vi "NoItemsFound.vi"(8 "error in (no error)":errorcluster, 11 "ExecuteMultipleBuildSpecs in":refnum<class "ExecuteMultipleBuildSpecs.lvclass">) -> (2 "CLI Process Return Code":i32, 3 "ExecuteMultipleBuildSpecs out":refnum<class "ExecuteMultipleBuildSpecs.lvclass">)   [LabVIEW 2020, in "ExecuteMultipleBuildSpecs.lvclass"]
doc: "Sets the LabVIEWCLI exit code if no build specs matching the criteria are found in the project."
uses:
  ExecuteMultipleBuildSpecs.lvclass
  Program Files (x86)/National Instruments/Shared/LabVIEW CLI/Operations/CoreOperation/CoreOperation.lvclass
  Program Files (x86)/National Instruments/Shared/LabVIEW CLI/Operations/Utilities/Logger/Logger.lvclass
  C:/Program Files (x86)/National Instruments/Shared/LabVIEW CLI/Operations/CoreOperation/CoreOperation.lvclass
  C:/Work/1_New Activities/JenkinsTest/BuildSystem/lv/operations/ExecuteMultipleBuildSpecs/ExecuteMultipleBuildSpecs.lvclass
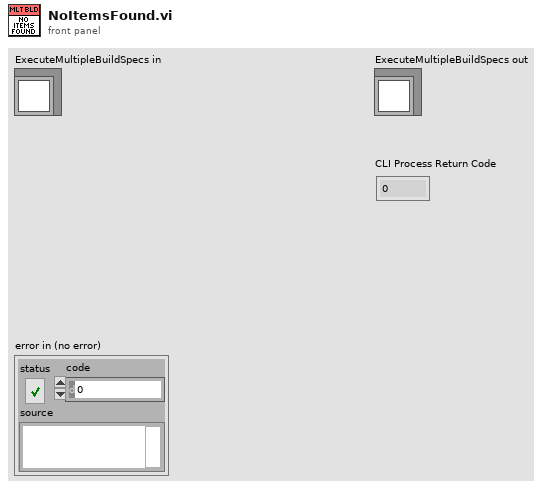
[diagram p1: front panel]
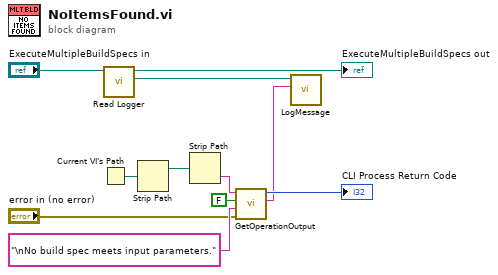
[diagram p0: block diagram]
diagram:
  n1 = Current VI's Path() -> (path=w9:path)
  n2 = call "Read Logger.vi"("CoreOperation in"="ExecuteMultipleBuildSpecs in") -> ("Logger.lvclass"=w2:refnum<class "Logger.lvclass">, "CoreOperation out"=→"ExecuteMultipleBuildSpecs out":refnum<class "ExecuteMultipleBuildSpecs.lvclass">)  [unwired: 8 in, 1 out]
  n3 = Strip Path(path=w9) -> (stripped path=w8:path)  [unwired: 1 out]
  n4 = Strip Path(path=w8) -> (name=w7:string)  [unwired: 1 out]
  n5 = call "GetOperationOutput.vi"("error in (no error)"="error in (no error)", "Operation Output/Error In"="\nNo build spec meets input parameters." ("format string"), "Operation succeeded?"=FALSE, "Operation Name"=w7) -> ("Operation Output/Error Out"=w1:string, "CLI Process Return Code"=→"CLI Process Return Code":i32)  [unwired: 6 in]
  n6 = call "LogMessage.vi"("Message"=w1, "Logger in"=w2) -> ()  [unwired: 8 in, 2 out]
